vi "Configure Calibration Kit.vi"(7 "Connector type":T1(ring), 8 "error in (no error)":errorcluster, 10 "Cal kit Name":string, 11 "VNA-Keysight PNA in":refnum<class "VNA-Keysight PNA.lvclass">) -> (0 "error out":errorcluster, 3 "VNA-Keysight PNA out":refnum<class "VNA-Keysight PNA.lvclass">)   [LabVIEW 2020, in "VNA-Keysight PNA.lvclass"]
doc: "Configure the calibration kit to use."
uses:
  VNA-Keysight PNA.lvclass
  C:/Sandbox/Git_Sandbox/WiSpry Test Framework source code (LV20)/WiSpry Test Framework/Instruments/Instrument.lvclass
  Instrument.lvclass/Instrument.ctl
  Instrument.lvclass
  <instrlib>/Keysight PNA Series/Keysight PNA Series.lvlib
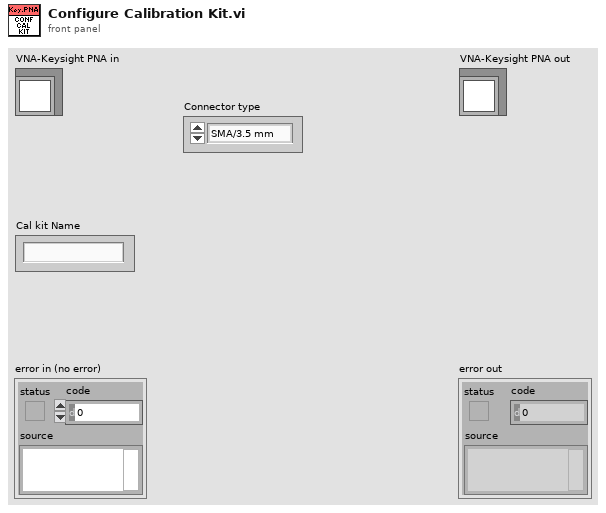
[diagram p1: front panel]
types:
  T1 = enum16{"SMA/3.5 mm", "2.92 mm", "2.4 mm", "1.85 mm", "N 50 Ohm", "N 75 Ohm", "7-16"}
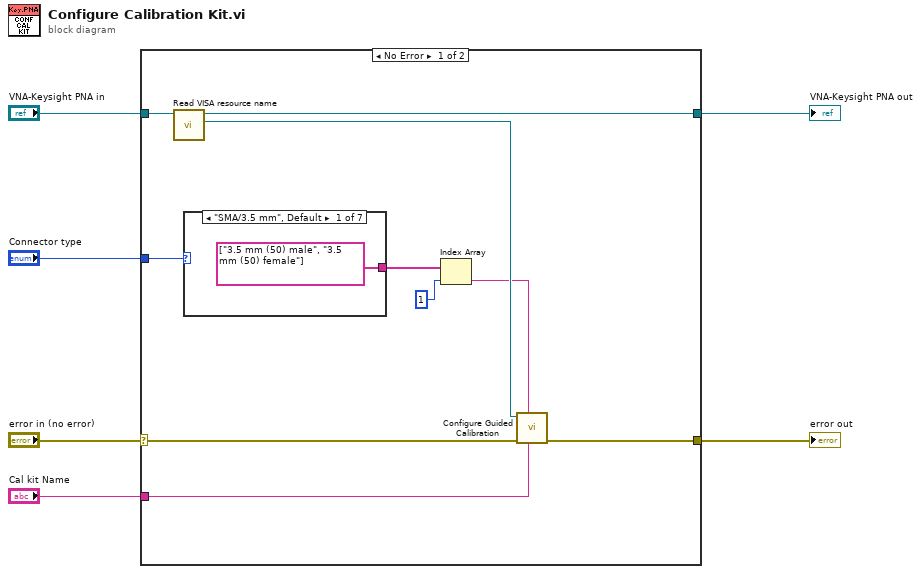
[diagram p0: block diagram]
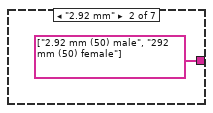
[diagram p2: hidden frame]
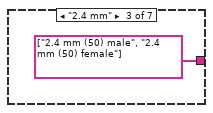
[diagram p3: hidden frame]
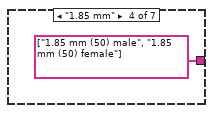
[diagram p4: hidden frame]
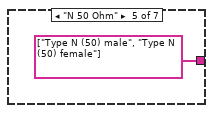
[diagram p5: hidden frame]
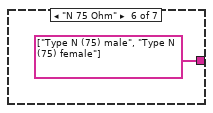
[diagram p6: hidden frame]
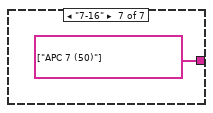
[diagram p7: hidden frame]
diagram:
  n1 = case shown="No Error" "error in (no error)" {
    selector: "error in (no error)" -> [w14 w24]
    tunnel: [w15 w25] -> w4
    tunnel: "VNA-Keysight PNA in" -> [w16 w25]
    tunnel: [w12 w24] -> w5
    tunnel: "Cal kit Name" -> [w11 _]
    tunnel: "Connector type" -> [w10 _]
    frame No Error {
      n2 = call "Read VISA resource name.vi"("Instrument in"=w16) -> ("VISA resource name"=w13:refnum<visa-resource-name>, "Instrument out"=w15:refnum<class "VNA-Keysight PNA.lvclass">)  [unwired: 9 in]
      n3 = case shown="\"SMA/3.5 mm\", Default" w10 {
        tunnel: [string[] ["3.5 mm (50) male", "3.5 mm (50) female"] string[] ["2.92 mm (50) male", "292 mm (50) female"] string[] ["2.4 mm (50) male", "2.4 mm (50) female"] string[] ["1.85 mm (50) male", "1.85 mm (50) female"] string[] ["Type N (50) male", "Type N (50) female"] string[] ["Type N (75) male", "Type N (75) female"] string[] ["APC 7 (50)"]] -> w9
        frame "SMA/3.5 mm", Default {
        }
        frame "2.92 mm" {
        }
        frame "2.4 mm" {
        }
        frame "1.85 mm" {
        }
        frame "N 50 Ohm" {
        }
        frame "N 75 Ohm" {
        }
        frame "7-16" {
        }
      }
      n4 = Index Array(array=w9, index=1) -> (element=w7:string)
      n5 = call <instrlib>:"Configure Guided Calibration.vi"("Calibration Kit (\"\")"=w11, "Connector (\"Not used\")"=w7, "error in (no error)"=w14, "VISA resource name"=w13) -> ("error out"=w12:errorcluster)  [unwired: 6 in, 1 out]
    }
    frame Error {
    }
  }
  "error out" <- w5
  "VNA-Keysight PNA out" <- w4
